vi "HiFiveUnmatched_GetSamplingRate.vi"(11 "Channel Configuration":T1[](array[typedef])) -> (3 "Sampling Rate":dbl)   [LabVIEW 2020]
uses:
  HiFiveUnmatched_PowerLineCfg.ctl
  7da1212d-d809-4a7f-8d6c-b93c896aa850.vi
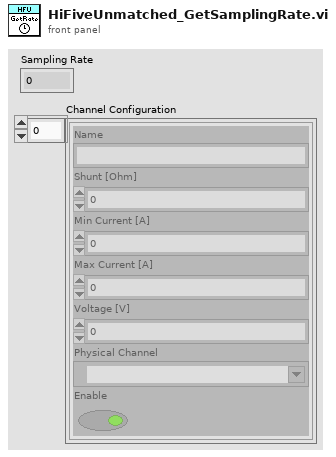
[diagram p1: front panel]
types:
  T1 = typedef "HiFiveUnmatched_PowerLineCfg.ctl" = cluster{"Name":string, "Shunt [Ohm]":dbl, "Min Current [A]":dbl, "Max Current [A]":dbl, "Voltage [V]":dbl, "Physical Channel":tag, "Enable":bool}
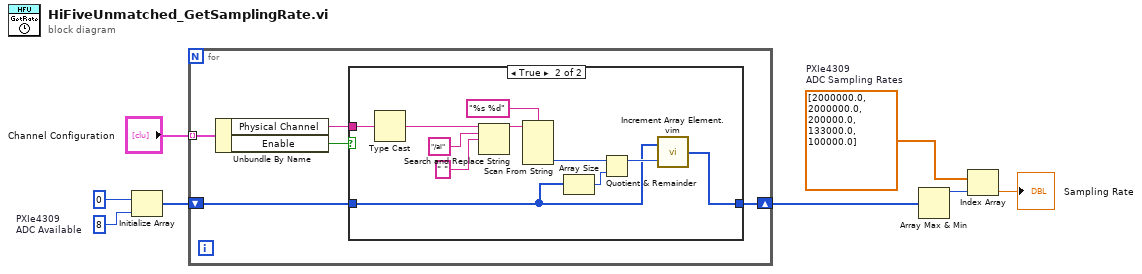
[diagram p0: block diagram]
diagram:
  w3 = dbl[] [2000000.0, 2000000.0, 200000.0, 133000.0, 100000.0]  # PXIe4309 ADC Sampling Rates
  w8 = 8  # PXIe4309 ADC Available
  n1 = Initialize Array(0 ("element"), w8) -> (w6:i32[])
  n2 = for {
    shift-right: [w12] -> w4
    shift-left: w6 -> [w13]
    tunnel: "Channel Configuration" -> [w11] mode=indexing
    n3 = Unbundle By Name(w11) -> ("Physical Channel"=w9:tag, "Enable"=w10:bool)
    n4 = case shown="True" w10 {
      tunnel: w13 -> [w14 w17]
      tunnel: [w14 w16] -> w12
      tunnel: w9 -> [_ w15]
      frame False {
      }
      frame True {
        n5 = Type Cast(x=w15) -> (*(type *) &x=w21:string)  [unwired: 1 in]
        n6 = Search and Replace String(input string=w21, search string="/ai", replace string=" " ("replace string (\"\")")) -> (result string=w20:string)  [unwired: 5 in, 3 out]
        n7 = Scan From String(format string="%s %d", input string=w20) -> (output 2=w24:i32)  [unwired: 5 in, 3 out]
        n8 = Array Size(array=w17) -> (size(s)=w18:i32)
        n9 = Quotient & Remainder(x=w24, y=w18) -> (x-y*floor(x/y)=w19:i32)  [unwired: 1 out]
        n10 = call "Increment Array Element.vim"("index"=w19, "array in"=w17) -> ("array out"=w16:i32[])
      }
    }
  }
  n11 = Array Max & Min(array=w4) -> (max value=w5:i32)  [unwired: 3 out]
  n12 = Index Array(array=w3, index=w5) -> (element=→"Sampling Rate":dbl)
